vi "SENS_CORR_COLL_GUID_ADAP_PATH.vi"(0 "VISA IN":refnum<visa-resource-name>, 1 "Adapter Index":i32, 2 "Port Pairs":string, 5 "error in":errorcluster, 7 "Channel":i32) -> (14 "VISA Out":refnum<visa-resource-name>, 19 "error out":errorcluster)   [LabVIEW 2018, in "PNA-X.lvlib"]
doc: "SENSe<cnum>:CORRection:COLLect:GUIDed:ADAPter<n>PATHs <port pairs> \n(Write-only) Specifies the port pairs for which the adapter will be used for a THRU connection. \nFor example, for a 3-port cal on channel 1 using ports 1,2,and 3), to use adapter 1 between the ports (1 \nto 2) and (1 to 3) the following command is used: SENS1:CORR:COLL:GUID:ADAP1:PATH \n1,2,1,3. \nThe adapter must have the same DUT connectors as the ports that are already specified for these ports. \nParameters \n<cnum> Any existing channel number. If unspecified, value is set to 1 \n<n> Adapter index number that was returned from \nSENS:CORR:COLL:GUID:ADAP:CREate? \n<port pair> Ports for which the adapter will be used. The orientation is not critical, as the \nPNA will align the connector types as necessary. The minimum number of \nThru connections required is the number of ports to calibrated -1. \nExamples See example using this command. \nQuery Syntax Not Applicable \nDefault Not Applicable \nSENSe:CORRection:COLLect:GUIDed:CKIT:PORT<pnum>:CATalog? \n1645\n\n(Read-only) Returns a comma-separated list of valid kits for each port. In addition to mechanical \ncalibration kits, this will include applicable characterizations found within ECal modules currently \nconnected to the PNA. \nIf two or more identical ECal modules are connected to the PNA, the returned list will include the \nserial numbers to distinguish the ECal modules. \nUse items in the list to select the kit to be used with the SENS:CORR:COLL:GUID:CKIT:PORT \ncommand. \nParameters \n<pnum> Any existing port number. If unspecified, value is set to 1 \nExamples SENS:CORR:COLL:GUID:CKIT:PORT1:CAT? \n'When \"Type N (50) male\" is specified for connector type, \nreturns: \n\"85054D, 85032F\" \n'When two identical ECal modules are connected for the connector \ntype, \n'the return string includes serial numbers \n\"85092-60010 ECal 10675, 85092-60010 ECal 00758\" \nReturn Type String \nDefault Not Applicable \nSENSe:CORRection:COLLect:GUIDed:CKIT:PORT<pnum>[:SELect] <kit> \n(Read-Write) Specifies the calibration kit for each port to be used during a guided calibration. An \nunused port does NOT need to have a specified Cal Kit. \nIf two or more identical ECal modules are connected to the PNA, the serial number must be included \nin the <kit> string to distinguish the ECal modules. See \nSENS:CORR:COLL:GUID:CKIT:PORT:CAT? \nNote: Sliding loads are not fully supported from Sens:Corr:Coll:Guided... The Measure button must \nbe manually pressed. \n1. Specify the connector type for the port with SENS:CORR:COLL:GUID:CONN:PORT. \n2. Query the valid available kits for the connector on each port with \nSENS:CORR:COLL:GUID:CKIT:PORT:CAT? \n1646\n\n3. Specify the kit using this command. \n4. Perform a query of this command. If the <kit> parameter was incorrectly entered, an error will be \nreturned.\nParameters \n<pnum> Any existing port number. If unspecified, value is set to 1 \n<kit> Calibration kit to be used for the specified port. \nExamples SENS:CORR:COLL:GUID:CKIT:PORT1 '85055A' \n'The following includes a serial number when two or more ECal \nmods are connected \nsense:correction:collect:guided:ckit:port2:select '85092-60010 \nECal 10685' \nQuery Syntax SENSe:CORRection:COLLect:GUIDed:CKIT:PORT<pnum>[:SELect]? \nReturn Type String - If the <kit> parameter was incorrectly entered while writing, an error \nwill be returned. \nDefault Not Applicable \nSENSe:CORRection:COLLect:GUIDed:CONNector:CATalog? \n(Read only) Returns a list of valid connectors based on the connector descriptions of the available cal \nkits. Use an item from the returned list to specify a connector for \nSENS:CORR:COLL:GUID:CONN:PORT \nExamples SENS:CORR:COLL:GUID:CONN:CAT? \nReturns: \nType N (50) female, Type N (50) male, APC 7 (50), 3.5 mm (50) \nmale, 3.5 mm (50) female, User Connector A \nReturn Type Comma separated string values \nDefault Not Applicable \nSENSe:CORRection:COLLect:GUIDed:CONNector:PORT<pnum>[:SELect] <conn> \n1647\n\n(Read-Write) Specifies a connector type for every port during the Guided Calibration procedure. Valid \nconnector names are stored within calibration kits. Some cal kits may include both male and female \nconnectors. Therefore, specifying connector gender may be required. \nThe PNA remembers previous Guided Cal settings. Therefore, for completeness, unused ports should \nbe defined as \"Not used\". See Guided Cal examples. \nA single port with a valid <conn> name indicates a 1-Port calibration will be performed. \nTwo ports with valid <conn> names indicate either a 2-Port SOLT or TRL calibration will be performed \ndepending on the standards definition found within the cal kit and the capability of the PNA. \nThree ports with valid <conn> names indicate a 3-Port calibration will be performed, and so forth. \nThe following steps could be followed to ensure port connectors are specified correctly: \nUse SENS:CORR:COLL:GUID:CONN:CAT? to query available connectors before specifying the port \nconnector. \n1. \nSelect a connector type using this command. 2. \nPerform a query of this command. If the <conn> parameter was incorrectly entered, an error will be \nreturned. \n3. \nSpecify the cal kit to use for each port with SENS:CORR:COLL:GUID:CKIT:PORT 4. \nParameters \n<pnum> Any existing port number. If unspecified, value is set to 1 \n<conn> String - DUT connector type to connect with PNA port <pnum> \nExamples 'Specifying a 2-port cal (1 & 2) on a 4-port PNA \nSENS:CORR:COLL:GUID:CONN:PORT1 'Type N (50) female' \nSENS:CORR:COLL:GUID:CONN:PORT2 'Type N (50) male' \nSENS:CORR:COLL:GUID:CONN:PORT3 'Not Used' \nSENS:CORR:COLL:GUID:CONN:PORT4 'Not Used' \nQuery Syntax SENSe:CORRection:COLLect:GUIDed:CONNector:PORT<pnum>[:SELect]? \nReturn Type String \nDefault Not Applicable \nSENSe:CORRection:COLLect:GUIDed:DESCription? <step> \n1648\n\n(Read-only) Returns the connection description for the specified calibration step. \nParameters \n<step> A number from 1 to the number of steps required to complete the calibration \n(Use SENS:CORR:COLL:GUID:STEP? to query the number of steps ) \nExamples SENS:CORR:COLL:GUID:DESC? 10 \n'Returns: \nConnect APC 7 Open to port3 \nReturn Type String \nDefault Not Applicable \nSENSe:CORRection:COLLect:GUIDed:DMATch:APPLy[:IMMediate] [<CalSetGUID>] \n(Write-only) Specifies a Cal Set as a source of delta match correction. \nIf CalSetGUID is not specified, then the Global Delta Match Cal Set is assumed. An error is returned \nif the specified Cal Set does not meet the following Delta Match criteria. The Global Delta Match Cal \ncan ALWAYS be applied. \nMust have been performed using ECal or as a guided mechanical cal (not Unguided). \nMust have the same start freq, stop freq, and number of points as the channel being calibrated. \nMust calibrate the ports that are required by the TRL or Unknown Thru cal as indicated by \nSENS:CORR:COLL:GUID:DMATch:APPLy:PORTs?. \nLearn more about Delta match calibration. \nSee example of a complete Delta Match calibration. \nParameters \n<CalSetGUID> Optional. GUID of the Cal Set to use. If unspecified, the Global Delta Match \nCal Set is used. \nExamples SENS:CORR:COLL:GUID:DMAT:APPL \nsense:correction:collect:guided:dmatch:apply:immediate \n\"{2B893E7A-971A-11d5-8D6C-00108334AE96}\" \nQuery Syntax Not Applicable \nDefault Not Applicable \nSENSe:CORRection:COLLect:GUIDed:DMATch:APPLy:PORTs? \n1649\n\n(Read-only) Returns the port numbers for which delta match correction is required. 0 (zero) is \nreturned if the Cal does NOT require Delta Match correction for one of the following reasons: \nThe Cal does NOT involve Unknown THRU or TRL. You specify this using \nSENS:CORR:COLL:GUID:METH <UNKN | TRL>. \nThe Cal DOES involve Unknown THRU or TRL, but the delta match data can be calculated by the Unknown \nThru or TRL Cal. Learn how this is possible. However, you can force the Cal to use the Delta Match data \nfrom a Cal Set. \nLearn more about Delta match calibration. \nSee example of a complete Delta Match calibration. \nParameters \nExamples SENS:CORR:COLL:GUID:APPL:PORT? \n'Returns: \n1,2,3 \nReturn Type Numeric \nDefault Not Applicable \nSENSe:CORRection:COLLect:GUIDed:DMATch[:INITiate] <conn>,<cKit> \n(Write-only) Initiates a global delta match calibration. \nLearn more about Global Delta Match calibration. \nSee example of a complete Delta Match calibration. \nParameters \n<conn> String. Connector type for port 1. All other ports are set automatically. \n<cKit> String Cal Kit for all ports. If incorrectly entered while writing, an error is \nreturned. \nExamples SENS:CORR:COLL:GUID:DMAT APC 3.5 female,\"85052B\" \nQuery Syntax Not Applicable \nDefault Not Applicable \nSENSe:CORRection:COLLect:GUIDed:ETERms:LOAD[:CSET] <cset>,<calPort> [,csPort] \n1650\n\n(Write-only) Loads 1-port error terms from a Cal Set into the current Guided Cal sequence. When the \nCal steps are recomputed, connection steps are removed due to the loading of the error terms. \nSee example of how to use this command. \nParameters \n<cset> String Name of User Cal Set in which the error terms reside. \n<pnum> Integer Port number of the current cal to receive error terms. \n[csPort] Integer Optional argument. Port number associated with the error terms in the \nCal Set. If unspecified, the same port number as <calPort> is used. \nExamples See example \nQuery Syntax Not Applicable \nDefault Not Applicable"
uses:
  PNA-X.lvlib
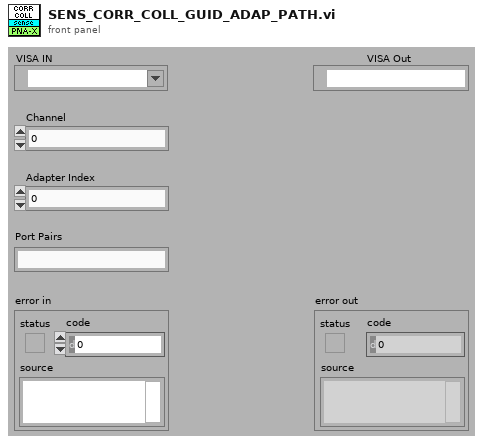
[diagram p1: front panel]
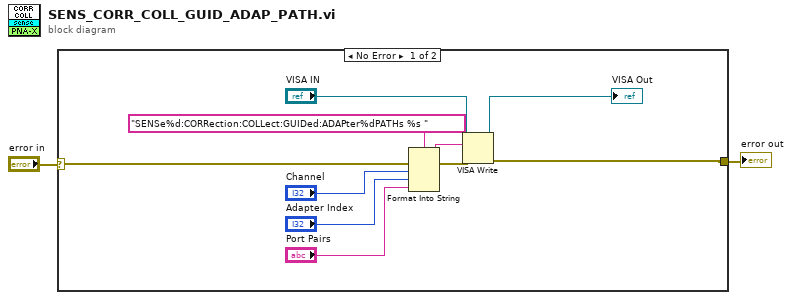
[diagram p0: block diagram]
diagram:
  n1 = case shown="No Error" "error in" {
    selector: "error in" -> [w12 w13]
    tunnel: [w7 w13] -> w1
    frame No Error {
      n2 = Format Into String(format string="SENSe%d:CORRection:COLLect:GUIDed:ADAPter%dPATHs %s " ("Cmdline"), error in=w12, "Channel", "Adapter Index", "Port Pairs") -> (resulting string=w10:string, error out=w11:errorcluster)  [unwired: 1 in]
      n3 = VISA Write(VISA resource name="VISA IN", write buffer=w10, error in (no error)=w11) -> (VISA resource name out=→"VISA Out":refnum<visa-resource-name>, error out=w7:errorcluster)  [unwired: 1 out]
    }
    frame Error {
    }
  }
  "error out" <- w1
